vi "Get Alarm Status.vi"(8 "error in (no error)":errorcluster, 11 "data":waveform(dbl)[](array[waveform])) -> (0 "error out":errorcluster, 3 "Alarms":T1)   [LabVIEW 2026, in "Acquisition.lvlib"]
uses:
  Acquisition.lvlib
  Alarms.ctl
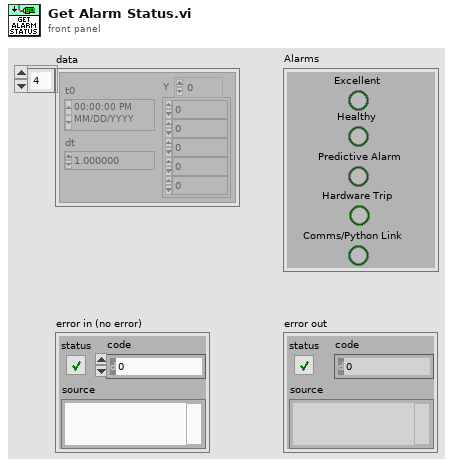
[diagram p1: front panel]
types:
  T1 = typedef "Alarms.ctl" = cluster{"Excellent":bool, "Healthy":bool, "Predictive Alarm":bool, "Hardware Trip":bool, "Comms/Python Link":bool}
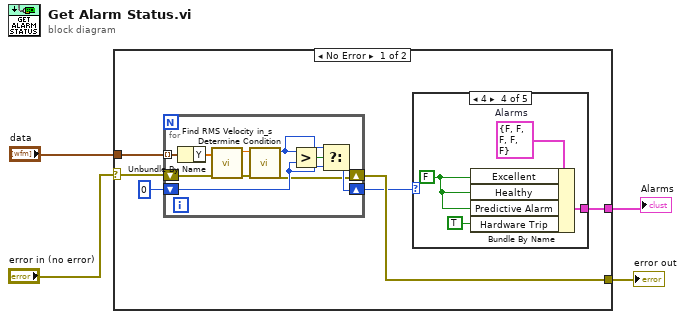
[diagram p0: block diagram]
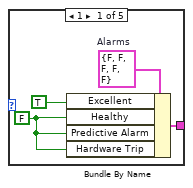
[diagram p2: hidden frame]
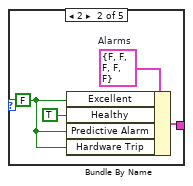
[diagram p3: hidden frame]
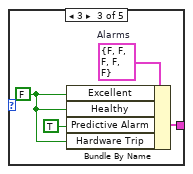
[diagram p4: hidden frame]
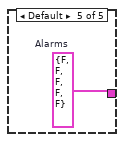
[diagram p5: hidden frame]
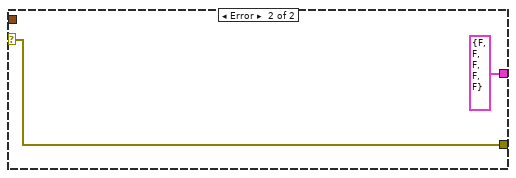
[diagram p6: hidden frame]
diagram:
  n1 = case shown="No Error" "error in (no error)" {
    selector: "error in (no error)" -> [w5 w38]
    tunnel: [w10 w38] -> w4
    tunnel: "data" -> [w9 _]
    tunnel: [w6 T1 {"Excellent"=FALSE, "Healthy"=FALSE, "Predictive Alarm"=FALSE, "Hardware Trip"=FALSE, "Comms/Python Link"=FALSE} ("Alarms")] -> w2
    frame No Error {
      n2 = for {
        shift-right: [w16] -> w8
        shift-left: 0 ("Condition") -> [w15]
        tunnel: w9 -> [w13] mode=indexing
        shift-right: [w11] -> w10
        shift-left: w5 -> [w12]
        n3 = Unbundle By Name(w13) -> ("Y"=w20:dbl[])
        n4 = call "Find RMS Velocity in_s .vi"("error in (no error)"=w12, "Y"=w20) -> ("error out"=w19:errorcluster, "rms value"=w14:dbl)  [unwired: 8 in]
        n5 = call "Determine Condition.vi"("error in (no error)"=w19, "RMS"=w14) -> ("error out"=w11:errorcluster, "Condition"=w17:i32)  [unwired: 8 in]
        n6 = Greater?(x=w17, y=w15) -> (0:w18:bool)
        n7 = Select(t=w17, s=w18, f=w15) -> (s? t:f=w16:i32)
      }
      n8 = case shown="4" w8 {
        tunnel: [w23 w27 w31 w35 w37] -> w6
        frame 1 {
          w22 = FALSE ("Excellent")
          w24 = T1 {"Excellent"=FALSE, "Healthy"=FALSE, "Predictive Alarm"=FALSE, "Hardware Trip"=FALSE, "Comms/Python Link"=FALSE}  # Alarms
          n9 = Bundle By Name(cluster=w24, "Excellent"=TRUE ("Healthy"), "Healthy"=w22, "Predictive Alarm"=w22, "Hardware Trip"=w22) -> (w23:T1)
        }
        frame 2 {
          w26 = FALSE ("Excellent")
          w28 = T1 {"Excellent"=FALSE, "Healthy"=FALSE, "Predictive Alarm"=FALSE, "Hardware Trip"=FALSE, "Comms/Python Link"=FALSE}  # Alarms
          n10 = Bundle By Name(cluster=w28, "Excellent"=w26, "Healthy"=TRUE, "Predictive Alarm"=w26, "Hardware Trip"=w26) -> (w27:T1)
        }
        frame 3 {
          w30 = FALSE ("Excellent")
          w32 = T1 {"Excellent"=FALSE, "Healthy"=FALSE, "Predictive Alarm"=FALSE, "Hardware Trip"=FALSE, "Comms/Python Link"=FALSE}  # Alarms
          n11 = Bundle By Name(cluster=w32, "Excellent"=w30, "Healthy"=w30, "Predictive Alarm"=TRUE ("Healthy"), "Hardware Trip"=w30) -> (w31:T1)
        }
        frame 4 {
          w33 = FALSE ("Excellent")
          w36 = T1 {"Excellent"=FALSE, "Healthy"=FALSE, "Predictive Alarm"=FALSE, "Hardware Trip"=FALSE, "Comms/Python Link"=FALSE}  # Alarms
          n12 = Bundle By Name(cluster=w36, "Excellent"=w33, "Healthy"=w33, "Predictive Alarm"=w33, "Hardware Trip"=TRUE ("Healthy")) -> (w35:T1)
        }
        frame Default {
          w37 = T1 {"Excellent"=FALSE, "Healthy"=FALSE, "Predictive Alarm"=FALSE, "Hardware Trip"=FALSE, "Comms/Python Link"=FALSE}  # Alarms
        }
      }
    }
    frame Error {
    }
  }
  "error out" <- w4
  "Alarms" <- w2
